vi "new alignment.vi"() -> ()   [LabVIEW 2010]
uses:
  <vilib>/Utility/inputDevices.llb/closeKeyboard.vi
  <vilib>/Utility/inputDevices.llb/keyboardAcquire.vi
panel:
  out "keys pressed":T1(array[ring])
  in  "Motor GPIB":u8=6 max=32 step=1 format="%#.0f"
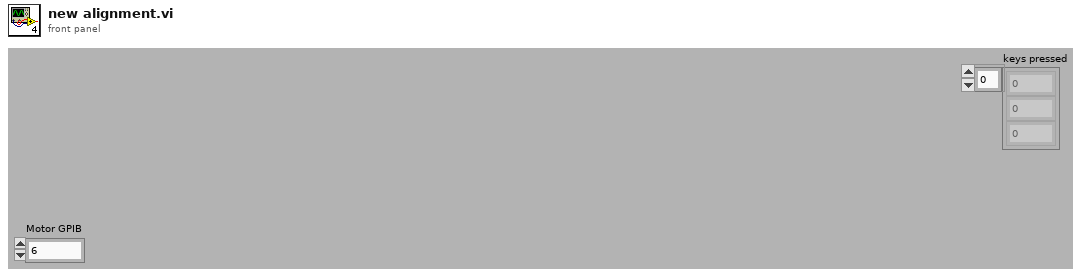
[diagram p1: front panel]
types:
  T1 = enum16{"0", "1", "2", "3", "4", "5", "6", "7", "8", "9", "A", "B", "C", "D", "E", "F", "G", "H", "I", "J", "K", "L", "M", "N", "O", "P", "Q", "R", "S", "T", "U", "V", "W", "X", "Y", "Z", "F1", "F2", "F3", "F4", "F5", "F6", "F7", "F8", "F9", "F10", "F11", "F12", "F13", "F14", "F15", "ADD", "BACK", "BACKSLASH", "CAPITAL", "COMMA", "DECIMAL", "DELETE", "DIVIDE", "DOWN", "END", "EQUALS", "ESCAPE", "GRAVE (`)", "HOME", "INSERT", "LBRACKET", "LCONTROL", "LEFT", "L ALT", "LSHIFT", "LWIN", "MINUS", "MULTIPLY", "NEXT", "NUMLOCK", "NUMPAD_0", "NUMPAD_1", "NUMPAD_2", "NUMPAD_3", "NUMPAD_4", "NUMPAD_5", "NUMPAD_6", "NUMPAD_7", "NUMPAD_8", "NUMPAD_9", "PAUSE", "PERIOD", "PRIOR (PG UP)", "RBRACKET", "RCONTROL", "RETURN", "RIGHT", "R ALT", "RSHIFT", "RWIN", "SCROLL", "SEMICOLON", "SLASH", "SPACE", "SUBTRACT", "TAB", "UP", "ENTER (num pad)", "' (quote)"}[]
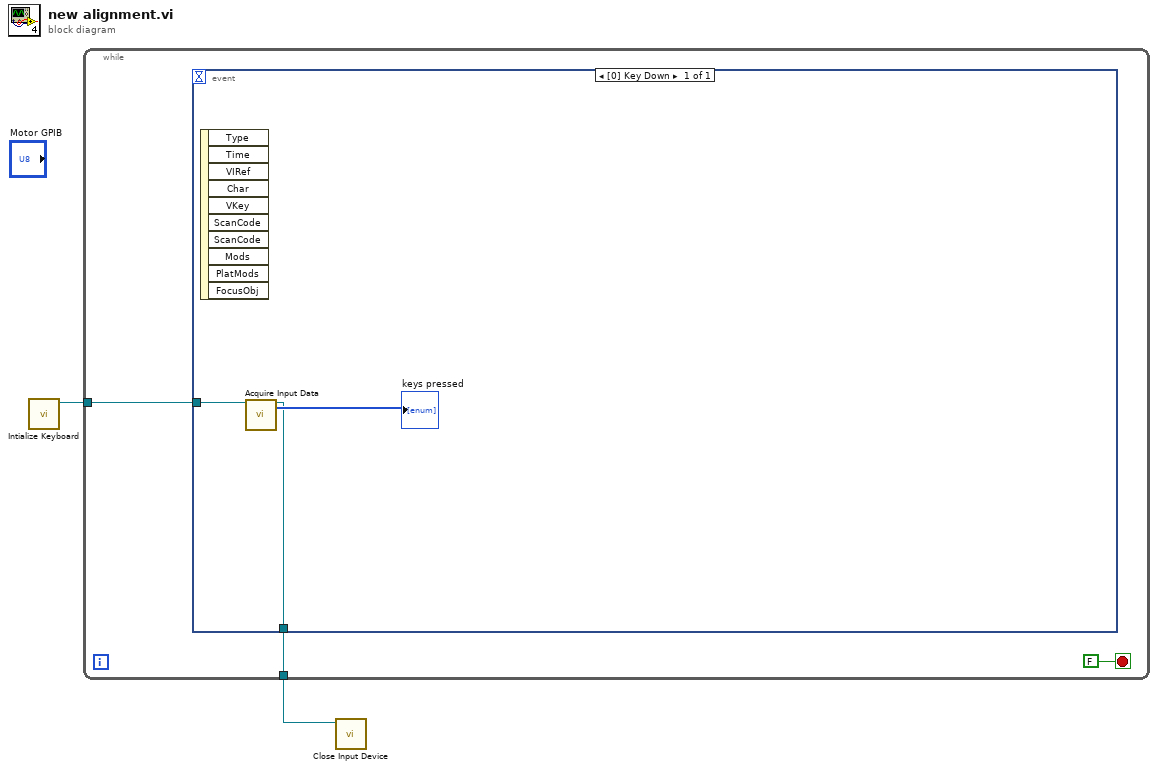
[diagram p0: block diagram]
diagram:
  n1 = call <vilib>:"Intialize Keyboard.vi"() -> ("device ID"=w2:refnum<k1>)  [unwired: 10 in, 1 out]
  n2 = while {
    tunnel: w2 -> [w4]
    tunnel: [w3] -> w1
    stop <- FALSE stop-if-true
    n3 = event shown="[0] Key Down" {
      selector: _ -> [_]
      dyn-events: _ -> [_]
      timeout: _ -> [_]
      tunnel: w4 -> [w8]
      tunnel: [w6] -> w3
      event Key Down {
        n4 = event-data() -> ()  [unwired: 1 in, 10 out]
        n5 = call-poly <vilib>:"Acquire Input Data.vi"("device ID"=w8) -> ("device ID"=w6:refnum<k1>, "keys pressed"=→"keys pressed":T1)  [unwired: 16 in, 1 out]
      }
    }
  }
  n6 = call-poly <vilib>:"Close Input Device.vi"("device ID"=w1) -> ()  [unwired: 9 in, 1 out]
